vi "Set Property.vi"(8 "error in (no error)":errorcluster, 9 "Value":dbl, 10 "Property":string, 11 "Gate in":refnum<class "Gate.lvclass">) -> (0 "error out":errorcluster, 3 "Gate out":refnum<class "Gate.lvclass">)   [LabVIEW 2020, in "Gate.lvclass"]
uses:
  Gate.lvclass
  Gate.lvclass/Gate.ctl
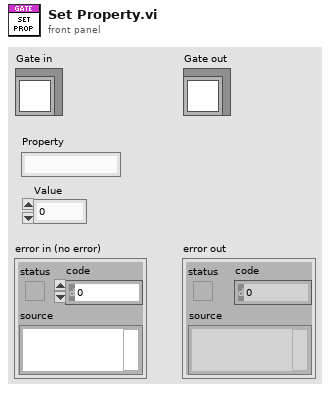
[diagram p1: front panel]
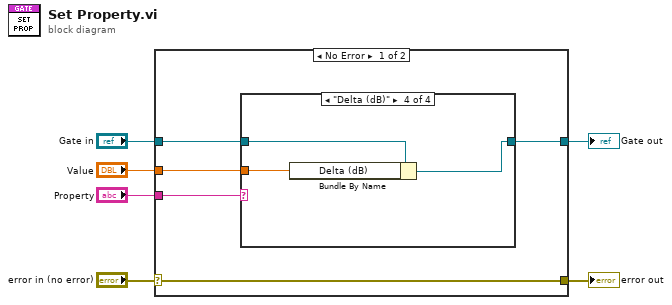
[diagram p0: block diagram]
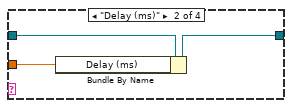
[diagram p3: hidden frame]
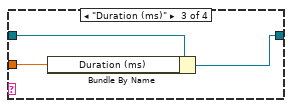
[diagram p4: hidden frame]
diagram:
  n1 = case shown="No Error" "error in (no error)" {
    selector: "error in (no error)" -> [w11 w23]
    tunnel: [w11 w23] -> w5
    tunnel: [w7 w22] -> w3
    tunnel: "Gate in" -> [w10 w22]
    tunnel: "Property" -> [w9 _]
    tunnel: "Value" -> [w8 _]
    frame No Error {
      n2 = case shown="\"Delta (dB)\"" w9 {
        tunnel: w10 -> [w12 w15 w18 w21]
        tunnel: w8 -> [_ w14 w17 w20]
        tunnel: [w12 w13 w16 w19] -> w7
        frame "False", Default {
        }
        frame "Delay (ms)" {
          n3 = Bundle By Name(cluster=w15, "Delay (ms)"=w14) -> (w13:refnum<class "Gate.lvclass">)
        }
        frame "Duration (ms)" {
          n4 = Bundle By Name(cluster=w18, "Duration (ms)"=w17) -> (w16:refnum<class "Gate.lvclass">)
        }
        frame "Delta (dB)" {
          n5 = Bundle By Name(cluster=w21, "Delta (dB)"=w20) -> (w19:refnum<class "Gate.lvclass">)
        }
      }
    }
    frame Error {
    }
  }
  "error out" <- w5
  "Gate out" <- w3
